vi "Make AtoD Channel Parameters.vi"(7 "DAQmx Device Name":tag="Dev1", 9 "A/D Pages":i32[](array[numeric]), 10 "CalData":T1(array[cluster])=[{"PageTitle"="PCI-6229 Digital Out Chls 0-7 DOUT", "NumLines"=8, "ChlNum"=["0", "1", "2", "3", "4", "5", "6", "7"], "ChlDesc"=["SO1 - Drive HPU Motor Starter", "SO2 - Drive Hyd Pressure Solenoid", "SO3 - Load HPU Motor Starter", "SO4 - Load Hyd Pressure Solenoid", "SO5 - TAVC Hi Speed Retract (J1)", "SO6 - TAVC Hi Spd Emer Retract (J2)", "SO7 - TAVC Hi Speed Retract (J3)", "SO8 - TAVC Hi Spd Emer Retract (J4)"], "ChlUnits"=["DOUT", "DOUT", "DOUT", "DOUT", "DOUT", "DOUT", "DOUT", "DOUT"], "ChlZero"=[0.0, 0.0, 0.0, 0.0, 0.0, 0.0, 0.0, 0.0], "ChlFactor"=[1.0, 1.0, 1.0, 1.0, 1.0, 1.0, 1.0, 1.0], "ChlConfig"=[12, 12, 12, 12, 12, 12, 12, 12]}, {"PageTitle"="PCI-6229 Digital Out Chls 8-15 DOUT", "NumLines"=8, "ChlNum"=["8", "9", "10", "11", "12", "13", "14", "15"], "ChlDesc"=["SO9 - TAVC Supply Shutoff (J1)", "SO10 - TAVC Supply Shutoff (J2)", "SO11 - TAVC Comp Force Select (J1)", "SO12 - TAVC Comp Force Select (J3)", "SO13 - TAVC Tension Force Select (J1)", "SO14 - TAVC Tension Force Select (J3)", "SO15 - Fixture Drive Extend Solenoid", "SO16 - Fixture Drive Retract Solenoid"], "ChlUnits"=["DOUT", "DOUT", "DOUT", "DOUT", "DOUT", "DOUT", "DOUT", "DOUT"], "ChlZero"=[0.0, 0.0, 0.0, 0.0, 0.0, 0.0, 0.0, 0.0], "ChlFactor"=[1.0, 1.0, 1.0, 1.0, 1.0, 1.0, 1.0, 1.0], "ChlConfig"=[12, 12, 12, 12, 12, 12, 12, 12]}, {"PageTitle"="PCI-6229 Digital Out Chls 16-23 DOUT", "NumLines"=8, "ChlNum"=["16", "17", "18", "19", "20", "21", "22", "23"], "ChlDesc"=["SO17 - Fixture High Speed Solenoid", "<spare>", "<spare>", "<spare>", "<spare>", "<spare>", "<spare>", "<spare>"], "ChlUnits"=["DOUT", "DOUT", "DOUT", "DOUT", "DOUT", "DOUT", "DOUT", "DOUT"], "ChlZero"=[0.0, 0.0, 0.0, 0.0, 0.0, 0.0, 0.0, 0.0], "ChlFactor"=[1.0, 1.0, 1.0, 1.0, 1.0, 1.0, 1.0, 1.0], "ChlConfig"=[12, 12, 12, 12, 12, 12, 12, 12]}, {"PageTitle"="PCI-6229 Digital In Chls 24-31 DIN", "NumLines"=8, "ChlNum"=["24", "25", "26", "27", "28", "29", "30", "31"], "ChlDesc"=["SI1 - TU IDS Extend Chl 1 Lim Swch", "SI2 - TU IDS Extend Chl 2 Lim Swch", "SI3 - TU IDS Retract Chl 1 Lim Swch", "SI4 - TU IDS Retract Chl 2 Lim Swch ", "SI5 - Load HPU Reservoir Fluid Level", "<spare>", "<spare>", "<spare>"], "ChlUnits"=["DIN", "DIN", "DIN", "DIN", "DIN", "DIN", "DIN", "DIN"], "ChlZero"=[0.0, 0.0, 0.0, 0.0, 0.0, 0.0, 0.0, 0.0], "ChlFactor"=[1.0, 1.0, 1.0, 1.0, 1.0, 1.0, 1.0, 1.0], "ChlConfig"=[11, 11, 11, 11, 11, 11, 11, 11]}, {"PageTitle"="PCI-6229 Digital In Chls 31-39 DIN", "NumLines"=8, "ChlNum"=["32", "33", "34", "35", "36", "37", "38", "39"], "ChlDesc"=["<spare>", "<spare>", "<spare>", "<spare>", "<spare>", "<spare>", "<spare>", "<spare>"], "ChlUnits"=["DIN", "DIN", "DIN", "DIN", "DIN", "DIN", "DIN", "DIN"], "ChlZero"=[0.0, 0.0, 0.0, 0.0, 0.0, 0.0, 0.0, 0.0], "ChlFactor"=[1.0, 1.0, 1.0, 1.0, 1.0, 1.0, 1.0, 1.0], "ChlConfig"=[11, 11, 11, 11, 11, 11, 11, 11]}, {"PageTitle"="PCI-6229 Counter In Chls 40-47 CTR", "NumLines"=8, "ChlNum"=["40", "41", "42", "43", "44", "45", "46", "47"], "ChlDesc"=["PF8 - Fixture Chain Rotary Encoder A", "PF9 - Fixture Chain Rotary Encoder B", "PF10 - Fixture Chain Rotary Encoder Z", "<spare>", "<spare>", "<spare>", "<spare>", "<spare>"], "ChlUnits"=["DIN", "DIN", "DIN", "DIN", "DIN", "DIN", "DIN", "DIN"], "ChlZero"=[0.0, 0.0, 0.0, 0.0, 0.0, 0.0, 0.0, 0.0], "ChlFactor"=[1.0, 1.0, 1.0, 1.0, 1.0, 1.0, 1.0, 1.0], "ChlConfig"=[13, 13, 13, 13, 13, 13, 13, 13]}, {"PageTitle"="PCI-6229 Analog Out AOUT", "NumLines"=4, "ChlNum"=["0", "1", "2", "3"], "ChlDesc"=["AO1 - Fixture Chain Load Servovalve", "AO2 - TAVC Drive Speed Servovalve", "<spare>", "<spare>"], "ChlUnits"=["Volts", "Volts", "<none>", "<none>"], "ChlZero"=[0.0, 0.0, 0.0, 0.0], "ChlFactor"=[1.0, 1.0, 1.0, 1.0], "ChlConfig"=[1, 1, 1, 1]}, {"PageTitle"="PCI-6229 Analog In Chls 0-15 AIN", "NumLines"=16, "ChlNum"=["0", "1", "2", "3", "4", "5", "6", "7", "8", "9", "10", "11", "12", "13", "14", "15"], "ChlDesc"=["P1 - Drive Hyd Motor Extend Pressure", "P2 - Drive Hyd Motor Retract Pressure", "P3 - Load Hyd Motor Extend Pressure", "P4 - Load Hyd Motor Retract Pressure", "P5 - TAVC Pressure A (J1)", "P6 - TAVC Pressure A (J3)", "P7 - TAVC Pressure B (J1)", "P8 - TAVC Pressure B (J3)", "F1 - Drive Hydraulic Motor Flow Rate", "S2 - Test Unit Speed Sensor Chl 1", "S3 - Test Unit Speed Sensor Chl 2", "T1 - Fixture Torque Sensor", "PS2 - Test Unit Position Sensor Chl 1", "PS3 - Test Unit Position Sensor Chl 2", "TS1 - TAVC Temperature A RTD", "TS2 - TAVC Temperature B RTD"], "ChlUnits"=["psig", "psig", "psig", "psig", "psig", "psig", "psig", "psig", "gpm", "fps", "fps", "in-lbf", "in", "in", "Deg-F", "Deg-F"], "ChlZero"=[0.0, 0.0, 0.0, 0.0, 0.0, 0.0, 0.0, 0.0, 0.0, 0.0, 0.0, 0.0, 0.0, 0.0, 0.0, 0.0], "ChlFactor"=[300.0, 300.0, 500.0, 500.0, 300.0, 300.0, 300.0, 300.0, 3.0, 0.0, 1.0, 1.0, 700.0, 0.0, 0.0, 0.0], "ChlConfig"=[1, 1, 1, 1, 1, 1, 1, 1, 1, 1, 1, 1, 1, 1, 1, 1]}, {"PageTitle"="PCI-6229 Analog In Chls 16-31 AIN", "NumLines"=16, "ChlNum"=["16", "17", "18", "19", "20", "21", "22", "23", "24", "25", "26", "27", "28", "29", "30", "31"], "ChlDesc"=["<spare>", "<spare>", "<spare>", "<spare>", "<spare>", "<spare>", "<spare>", "<spare>", "<spare>", "<spare>", "<spare>", "<spare>", "<spare>", "<spare>", "<spare>", "<spare>"], "ChlUnits"=["<none>", "<none>", "<none>", "<none>", "<none>", "<none>", "<none>", "<none>", "<none>", "<none>", "<none>", "<none>", "<none>", "<none>", "<none>", "<none>"], "ChlZero"=[0.0, 0.0, 0.0, 0.0, 0.0, 0.0, 0.0, 0.0, 0.0, 0.0, 0.0, 0.0, 0.0, 0.0, 0.0, 0.0], "ChlFactor"=[0.0, 0.0, 0.0, 0.0, 0.0, 0.0, 0.0, 0.0, 0.0, 0.0, 0.0, 0.0, 0.0, 0.0, 0.0, 0.0], "ChlConfig"=[1, 1, 1, 1, 1, 1, 1, 1, 1, 1, 1, 1, 1, 1, 1, 1]}, {"PageTitle"="USB-9211 Module 1 Chls 0-3 T/C AIN", "NumLines"=4, "ChlNum"=["0", "1", "2", "3"], "ChlDesc"=["TC1 - Test Unit Gbx Housing 1 Temp", "TC2 - Test Unit Gbx Housing 2 Temp", "TC3 - Drive Hyd Reservoir Fluid Temp", "TC4 - Load Hyd Reservoir Fluid Temp"], "ChlUnits"=["Deg-F", "Deg-F", "Deg-F", "Deg-F"], "ChlZero"=[0.0, 0.0, 0.0, 0.0], "ChlFactor"=[1.0, 1.0, 1.0, 1.0], "ChlConfig"=[3, 3, 3, 3]}, {"PageTitle"="USB-9211 Module 2 Chls 4-7 T/C AIN", "NumLines"=4, "ChlNum"=["4", "5", "6", "7"], "ChlDesc"=["TC5 - Extra 1", "TC6 - Extra 2", "TC7 - Extra 3", "TC8 - Extra 4"], "ChlUnits"=["Deg-F", "Deg-F", "Deg-F", "Deg-F"], "ChlZero"=[0.0, 0.0, 0.0, 0.0], "ChlFactor"=[1.0, 1.0, 1.0, 1.0], "ChlConfig"=[3, 3, 3, 3]}] {"ChlFactor" format="%.3f"; "ChlZero" format="%.3f"}, 11 "A/D Active Chl List":i32[](array[numeric])) -> (0 "Chl Factors":dbl[](array[numeric]) format="%.2f", 1 "Chl Zeroes":dbl[](array[numeric]) format="%.2f", 2 "NI-DAQ A/D Chls":tag[](array[tag]), 3 "DAQmx Physical Channel Names":string, 4 "Chl Descriptions":string[](array[string]), 5 "NumChls":i32, 6 "DAQmx Chl Names":string[](array[string]))   [LabVIEW 2013]
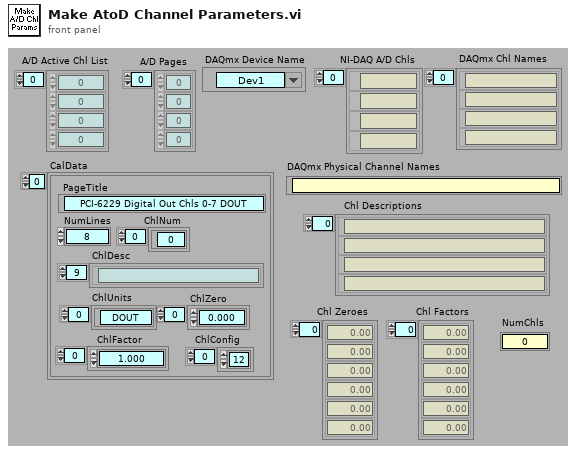
[diagram p1: front panel]
types:
  T1 = cluster{"PageTitle":string, "NumLines":i32, "ChlNum":string[], "ChlDesc":string[], "ChlUnits":string[], "ChlZero":sgl[], "ChlFactor":sgl[], "ChlConfig":u16[]}[]
  T2 = cluster{"PageTitle":string, "NumLines":i32, "ChlNum":string[], "ChlDesc":string[], "ChlUnits":string[], "ChlZero":sgl[], "ChlFactor":sgl[], "ChlConfig":u16[]}
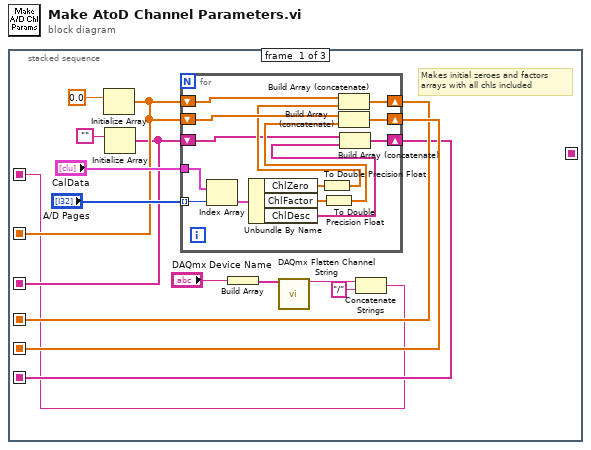
[diagram p0: block diagram]
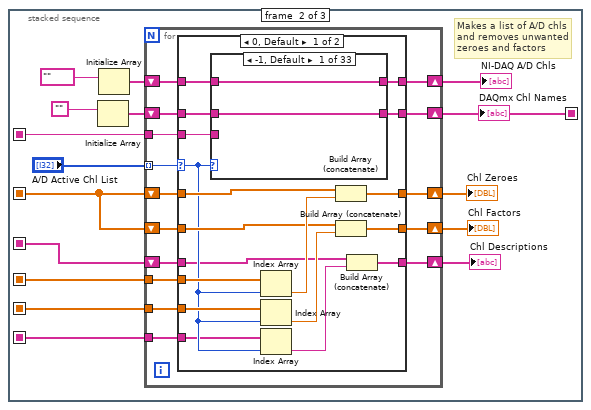
[diagram p2: hidden frame]
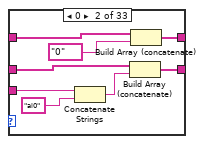
[diagram p3: hidden frame]
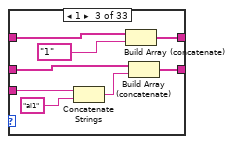
[diagram p4: hidden frame]
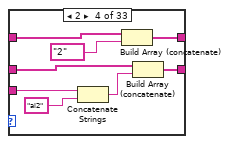
[diagram p5: hidden frame]
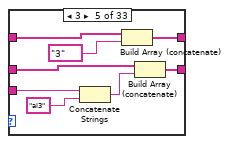
[diagram p6: hidden frame]
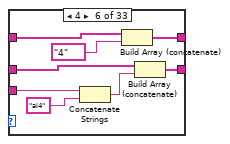
[diagram p7: hidden frame]
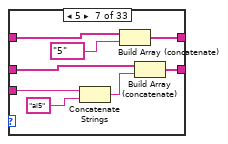
[diagram p8: hidden frame]
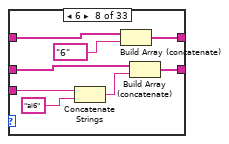
[diagram p9: hidden frame]
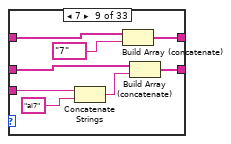
[diagram p10: hidden frame]
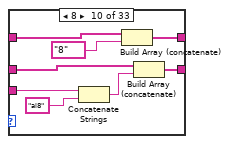
[diagram p11: hidden frame]
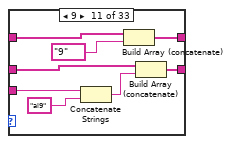
[diagram p12: hidden frame]
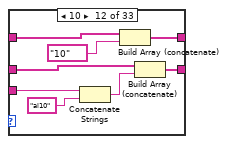
[diagram p13: hidden frame]
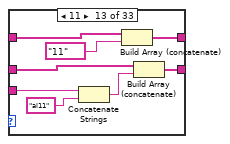
[diagram p14: hidden frame]
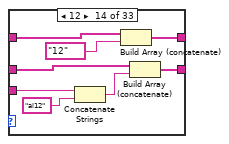
[diagram p15: hidden frame]
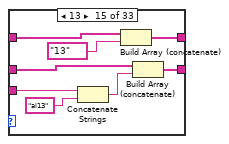
[diagram p16: hidden frame]
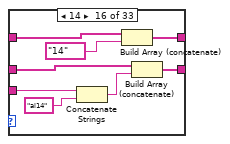
[diagram p17: hidden frame]
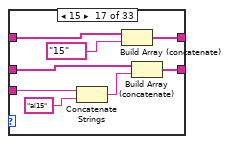
[diagram p18: hidden frame]
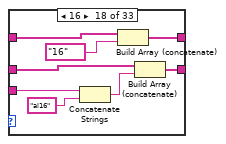
[diagram p19: hidden frame]
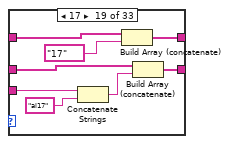
[diagram p20: hidden frame]
diagram:
  n1 = stacked-sequence {
    seq-local: [w11 _ _] -> [_ w40 _]
    seq-local: [w10 _ _] -> [_ w41 _]
    seq-local: [w9 _ _] -> [_ w39 _]
    seq-local: [w7 _ _] -> [_ w35 _]
    seq-local: [w6 _ _] -> [_ w36 _]
    seq-local: [w1 _ _] -> [_ w30 _]
    seq-local: [_ w29 _] -> [_ _ w342]
    frame #0 {
      # "Makes initial zeroes and factors\narrays with all chls included"
      n2 = Initialize Array(0.0) -> (w9:dbl[])  [unwired: 1 in]
      n3 = Initialize Array("") -> (w6:string[])  [unwired: 1 in]
      n4 = for {
        tunnel: "CalData" -> [w28]
        tunnel: "A/D Pages" -> [w27] mode=indexing
        shift-right: [w25] -> w10
        shift-left: w9 -> [w23]
        shift-right: [w22] -> w11
        shift-left: w9 -> [w21]
        shift-right: [w15] -> w7
        shift-left: w6 -> [w17]
        n5 = Index Array(array=w28, index=w27) -> (element=w26:T2)
        n6 = Unbundle By Name(w26) -> ("ChlZero"=w24:sgl[], "ChlFactor"=w20:sgl[], "ChlDesc"=w16:string[])
        n7 = To Double Precision Float(number=w24) -> (double precision float=w19:dbl[])
        n8 = To Double Precision Float(number=w20) -> (double precision float=w18:dbl[])
        n9 = Build Array (concatenate)(w23, w19) -> (w25:dbl[])
        n10 = Build Array (concatenate)(w21, w18) -> (w22:dbl[])
        n11 = Build Array (concatenate)(w17, w16) -> (w15:string[])
      }
      n12 = Build Array("DAQmx Device Name") -> (w4:tag[])
      n13 = call <vilib>:"DAQmx Flatten Channel String.vi"("names in"=w4) -> ("names out"=w3:string)  [unwired: 13 in, 1 out]
      n14 = Concatenate Strings(w3, "/" ("string")) -> (w1:string)
    }
    frame #1 {
      # "Makes a list of A/D chls\nand removes unwanted\nzeroes and factors"
      n15 = Initialize Array("") -> (w31:string[])  [unwired: 1 in]
      n16 = Initialize Array(tag "") -> (w42:tag[])  [unwired: 1 in]
      n17 = for {
        tunnel: "A/D Active Chl List" -> [w59] mode=indexing
        shift-right: [w57] -> w33
        shift-left: w42 -> [w58]
        shift-right: [w54] -> w38
        shift-left: w39 -> [w56]
        tunnel: w41 -> [w52]
        tunnel: w40 -> [w51]
        shift-right: [w53] -> w37
        shift-left: w39 -> [w55]
        shift-right: [w50] -> w34
        shift-left: w36 -> [w49]
        tunnel: w35 -> [w48]
        shift-right: [w47] -> w29
        shift-left: w31 -> [w46]
        tunnel: w30 -> [w45]
        n18 = case shown="0, Default" w59 {
          selector: w59 -> [w67 _]
          tunnel: w58 -> [w77 w340]
          tunnel: [w76 w340] -> w57
          tunnel: w56 -> [w74 w339]
          tunnel: w55 -> [w70 w338]
          tunnel: [w72 w339] -> w54
          tunnel: [w71 w338] -> w53
          tunnel: w52 -> [w75 _]
          tunnel: w51 -> [w69 _]
          tunnel: [w66 w337] -> w50
          tunnel: w49 -> [w65 w337]
          tunnel: w48 -> [w64 _]
          tunnel: [w62 w336] -> w47
          tunnel: w46 -> [w61 w336]
          tunnel: w45 -> [w60 _]
          frame 0, Default {
            n19 = case shown="-1, Default" w67 {
              tunnel: w77 -> [w79 w86 w94 w102 w110 w118 w126 w134 w142 w150 w158 w166 w174 w182 w190 w198 w206 w214 w222 w230 w238 w246 w254 w262 w270 w278 w286 w294 w302 w310 w318 w326 w334]
              tunnel: [w79 w85 w93 w101 w109 w117 w125 w133 w141 w149 w157 w165 w173 w181 w189 w197 w205 w213 w221 w229 w237 w245 w253 w261 w269 w277 w285 w293 w301 w309 w317 w325 w333] -> w76
              tunnel: [w78 w84 w90 w98 w106 w114 w122 w130 w138 w146 w154 w162 w170 w178 w186 w194 w202 w210 w218 w226 w234 w242 w250 w258 w266 w274 w282 w290 w298 w306 w314 w322 w330] -> w62
              tunnel: w61 -> [w78 w83 w89 w97 w105 w113 w121 w128 w136 w144 w152 w160 w168 w177 w184 w192 w200 w208 w216 w224 w232 w240 w248 w256 w264 w272 w280 w289 w296 w304 w312 w321 w328]
              tunnel: w60 -> [_ w82 w88 w96 w104 w112 w120 w129 w137 w145 w153 w161 w169 w176 w185 w193 w201 w209 w217 w225 w233 w241 w249 w257 w265 w273 w281 w288 w297 w305 w313 w320 w329]
              frame -1, Default {
              }
              frame 0 {
                n20 = Concatenate Strings(w82, "ai0") -> (w80:string)
                n21 = Build Array (concatenate)(w83, w80) -> (w84:string[])
                n22 = Build Array (concatenate)(w86, tag "0" ("channel (0)")) -> (w85:tag[])
              }
              frame 1 {
                n23 = Concatenate Strings(w88, "ai1") -> (w91:string)
                n24 = Build Array (concatenate)(w94, tag "1" ("channel (0)")) -> (w93:tag[])
                n25 = Build Array (concatenate)(w89, w91) -> (w90:string[])
              }
              frame 2 {
                n26 = Concatenate Strings(w96, "ai2") -> (w99:string)
                n27 = Build Array (concatenate)(w102, tag "2" ("channel (0)")) -> (w101:tag[])
                n28 = Build Array (concatenate)(w97, w99) -> (w98:string[])
              }
              frame 3 {
                n29 = Concatenate Strings(w104, "ai3") -> (w107:string)
                n30 = Build Array (concatenate)(w110, tag "3" ("channel (0)")) -> (w109:tag[])
                n31 = Build Array (concatenate)(w105, w107) -> (w106:string[])
              }
              frame 4 {
                n32 = Concatenate Strings(w112, "ai4") -> (w115:string)
                n33 = Build Array (concatenate)(w118, tag "4" ("channel (0)")) -> (w117:tag[])
                n34 = Build Array (concatenate)(w113, w115) -> (w114:string[])
              }
              frame 5 {
                n35 = Concatenate Strings(w120, "ai5") -> (w123:string)
                n36 = Build Array (concatenate)(w126, tag "5" ("channel (0)")) -> (w125:tag[])
                n37 = Build Array (concatenate)(w121, w123) -> (w122:string[])
              }
              frame 6 {
                n38 = Concatenate Strings(w129, "ai6") -> (w131:string)
                n39 = Build Array (concatenate)(w134, tag "6" ("channel (0)")) -> (w133:tag[])
                n40 = Build Array (concatenate)(w128, w131) -> (w130:string[])
              }
              frame 7 {
                n41 = Concatenate Strings(w137, "ai7") -> (w139:string)
                n42 = Build Array (concatenate)(w142, tag "7" ("channel (0)")) -> (w141:tag[])
                n43 = Build Array (concatenate)(w136, w139) -> (w138:string[])
              }
              frame 8 {
                n44 = Concatenate Strings(w145, "ai8") -> (w147:string)
                n45 = Build Array (concatenate)(w150, tag "8" ("channel (0)")) -> (w149:tag[])
                n46 = Build Array (concatenate)(w144, w147) -> (w146:string[])
              }
              frame 9 {
                n47 = Concatenate Strings(w153, "ai9") -> (w155:string)
                n48 = Build Array (concatenate)(w158, tag "9" ("channel (0)")) -> (w157:tag[])
                n49 = Build Array (concatenate)(w152, w155) -> (w154:string[])
              }
              frame 10 {
                n50 = Concatenate Strings(w161, "ai10") -> (w163:string)
                n51 = Build Array (concatenate)(w166, tag "10" ("channel (0)")) -> (w165:tag[])
                n52 = Build Array (concatenate)(w160, w163) -> (w162:string[])
              }
              frame 11 {
                n53 = Concatenate Strings(w169, "ai11") -> (w171:string)
                n54 = Build Array (concatenate)(w174, tag "11" ("channel (0)")) -> (w173:tag[])
                n55 = Build Array (concatenate)(w168, w171) -> (w170:string[])
              }
              frame 12 {
                n56 = Concatenate Strings(w176, "ai12") -> (w179:string)
                n57 = Build Array (concatenate)(w182, tag "12" ("channel (0)")) -> (w181:tag[])
                n58 = Build Array (concatenate)(w177, w179) -> (w178:string[])
              }
              frame 13 {
                n59 = Concatenate Strings(w185, "ai13") -> (w187:string)
                n60 = Build Array (concatenate)(w190, tag "13" ("channel (0)")) -> (w189:tag[])
                n61 = Build Array (concatenate)(w184, w187) -> (w186:string[])
              }
              frame 14 {
                n62 = Concatenate Strings(w193, "ai14") -> (w195:string)
                n63 = Build Array (concatenate)(w198, tag "14" ("channel (0)")) -> (w197:tag[])
                n64 = Build Array (concatenate)(w192, w195) -> (w194:string[])
              }
              frame 15 {
                n65 = Concatenate Strings(w201, "ai15") -> (w203:string)
                n66 = Build Array (concatenate)(w206, tag "15" ("channel (0)")) -> (w205:tag[])
                n67 = Build Array (concatenate)(w200, w203) -> (w202:string[])
              }
              frame 16 {
                n68 = Concatenate Strings(w209, "ai16") -> (w211:string)
                n69 = Build Array (concatenate)(w214, tag "16" ("channel (0)")) -> (w213:tag[])
                n70 = Build Array (concatenate)(w208, w211) -> (w210:string[])
              }
              frame 17 {
                n71 = Concatenate Strings(w217, "ai17") -> (w219:string)
                n72 = Build Array (concatenate)(w222, tag "17" ("channel (0)")) -> (w221:tag[])
                n73 = Build Array (concatenate)(w216, w219) -> (w218:string[])
              }
              frame 18 {
                n74 = Concatenate Strings(w225, "ai18") -> (w227:string)
                n75 = Build Array (concatenate)(w230, tag "18" ("channel (0)")) -> (w229:tag[])
                n76 = Build Array (concatenate)(w224, w227) -> (w226:string[])
              }
              frame 19 {
                n77 = Concatenate Strings(w233, "ai19") -> (w235:string)
                n78 = Build Array (concatenate)(w238, tag "19" ("channel (0)")) -> (w237:tag[])
                n79 = Build Array (concatenate)(w232, w235) -> (w234:string[])
              }
              frame 20 {
                n80 = Concatenate Strings(w241, "ai20") -> (w243:string)
                n81 = Build Array (concatenate)(w246, tag "20" ("channel (0)")) -> (w245:tag[])
                n82 = Build Array (concatenate)(w240, w243) -> (w242:string[])
              }
              frame 21 {
                n83 = Concatenate Strings(w249, "ai21") -> (w251:string)
                n84 = Build Array (concatenate)(w254, tag "21" ("channel (0)")) -> (w253:tag[])
                n85 = Build Array (concatenate)(w248, w251) -> (w250:string[])
              }
              frame 22 {
                n86 = Concatenate Strings(w257, "ai22") -> (w259:string)
                n87 = Build Array (concatenate)(w262, tag "22" ("channel (0)")) -> (w261:tag[])
                n88 = Build Array (concatenate)(w256, w259) -> (w258:string[])
              }
              frame 23 {
                n89 = Concatenate Strings(w265, "ai23") -> (w267:string)
                n90 = Build Array (concatenate)(w270, tag "23" ("channel (0)")) -> (w269:tag[])
                n91 = Build Array (concatenate)(w264, w267) -> (w266:string[])
              }
              frame 24 {
                n92 = Concatenate Strings(w273, "ai24") -> (w275:string)
                n93 = Build Array (concatenate)(w278, tag "24" ("channel (0)")) -> (w277:tag[])
                n94 = Build Array (concatenate)(w272, w275) -> (w274:string[])
              }
              frame 25 {
                n95 = Concatenate Strings(w281, "ai25") -> (w283:string)
                n96 = Build Array (concatenate)(w286, tag "25" ("channel (0)")) -> (w285:tag[])
                n97 = Build Array (concatenate)(w280, w283) -> (w282:string[])
              }
              frame 26 {
                n98 = Concatenate Strings(w288, "ai26") -> (w291:string)
                n99 = Build Array (concatenate)(w294, tag "26" ("channel (0)")) -> (w293:tag[])
                n100 = Build Array (concatenate)(w289, w291) -> (w290:string[])
              }
              frame 27 {
                n101 = Concatenate Strings(w297, "ai27") -> (w299:string)
                n102 = Build Array (concatenate)(w302, tag "27" ("channel (0)")) -> (w301:tag[])
                n103 = Build Array (concatenate)(w296, w299) -> (w298:string[])
              }
              frame 28 {
                n104 = Concatenate Strings(w305, "ai28") -> (w307:string)
                n105 = Build Array (concatenate)(w310, tag "28" ("channel (0)")) -> (w309:tag[])
                n106 = Build Array (concatenate)(w304, w307) -> (w306:string[])
              }
              frame 29 {
                n107 = Concatenate Strings(w313, "ai29") -> (w315:string)
                n108 = Build Array (concatenate)(w318, tag "29" ("channel (0)")) -> (w317:tag[])
                n109 = Build Array (concatenate)(w312, w315) -> (w314:string[])
              }
              frame 30 {
                n110 = Concatenate Strings(w320, "ai30") -> (w323:string)
                n111 = Build Array (concatenate)(w326, tag "30" ("channel (0)")) -> (w325:tag[])
                n112 = Build Array (concatenate)(w321, w323) -> (w322:string[])
              }
              frame 31 {
                n113 = Concatenate Strings(w329, "ai31") -> (w331:string)
                n114 = Build Array (concatenate)(w334, tag "31" ("channel (0)")) -> (w333:tag[])
                n115 = Build Array (concatenate)(w328, w331) -> (w330:string[])
              }
            }
            n116 = Index Array(array=w75, index=w67) -> (element=w73:dbl)
            n117 = Index Array(array=w69, index=w67) -> (element=w68:dbl)
            n118 = Index Array(array=w64, index=w67) -> (element=w63:string)
            n119 = Build Array (concatenate)(w74, w73) -> (w72:dbl[])
            n120 = Build Array (concatenate)(w70, w68) -> (w71:dbl[])
            n121 = Build Array (concatenate)(w65, w63) -> (w66:string[])
          }
          frame -1 {
          }
        }
      }
      "NI-DAQ A/D Chls" <- w33
      "Chl Zeroes" <- w38
      "Chl Factors" <- w37
      "Chl Descriptions" <- w34
      "DAQmx Chl Names" <- w29
    }
    frame #2 {
      # "Final values"
      n122 = Array Size(array=w342) -> (size(s)=→"NumChls":i32)
      n123 = call <vilib>:"DAQmx Flatten Channel String.vi"("names in"=w342) -> ("names out"=→"DAQmx Physical Channel Names":string)  [unwired: 13 in, 1 out]
    }
  }
